vi "CMD_Drive.vi"(1 "Line":string) -> (0 "Done":bool)   [LabVIEW 2016]
uses:
  Robot Global Data.vi
  <vilib>/addons/control/pid/pid.llb/PID (DBL).vi
  <vilib>/addons/control/pid/NI_PID_pid.lvlib
  Apple Gyro/Apple Pi Gyro Library.lvlib
panel:
  in  "Subcommands":string[](array[string])=["at", "at", "for", "to", "until"]
  in  "Parameters":i32[](array[numeric])=[1, 3, 3, 3, 1]
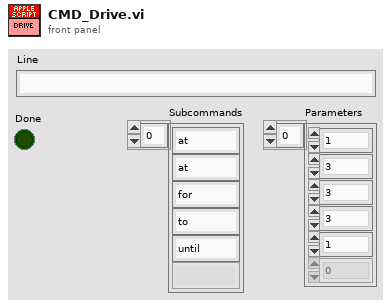
[diagram p1: front panel]
types:
  T1 = cluster{"proportional gain (Kc)":dbl, "integral time (Ti, min)":dbl, "derivative time (Td, min)":dbl}
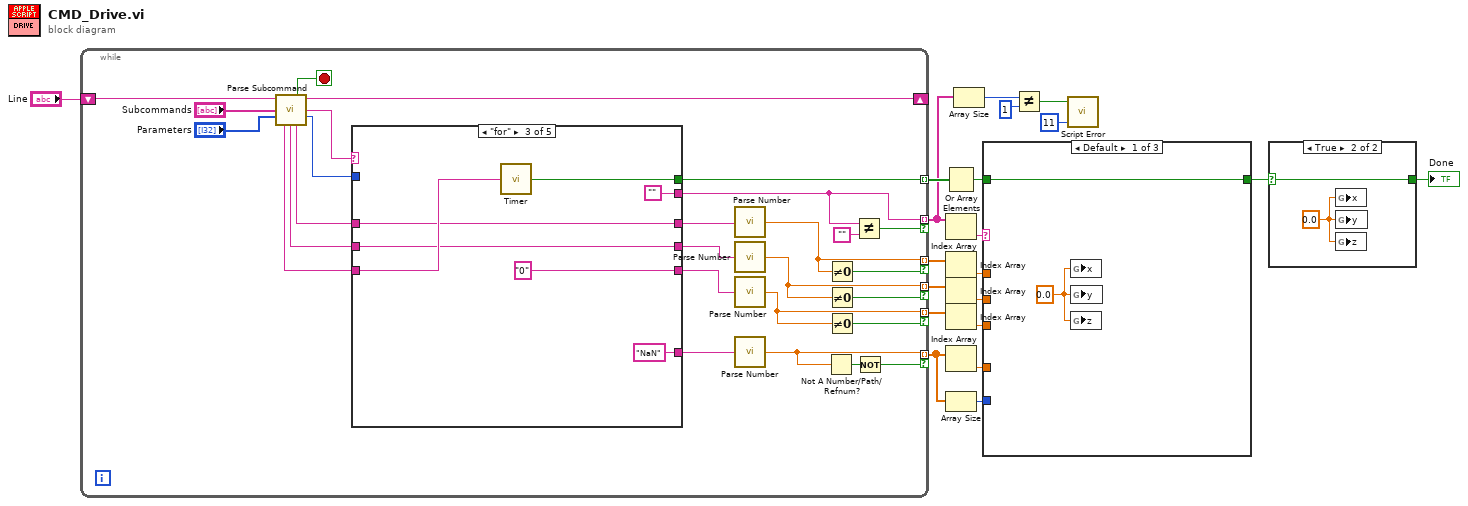
[diagram p0: block diagram]
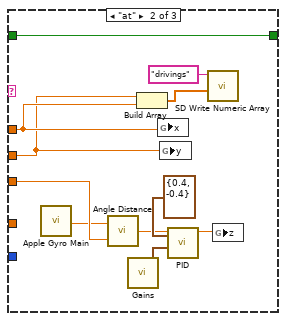
[diagram p3: hidden frame]
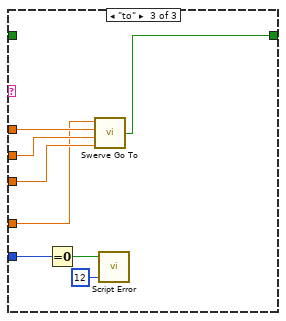
[diagram p4: hidden frame]
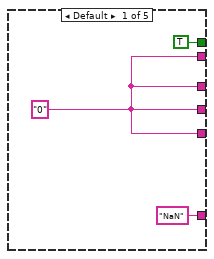
[diagram p5: hidden frame]
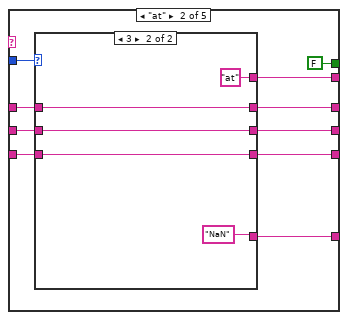
[diagram p6: hidden frame]
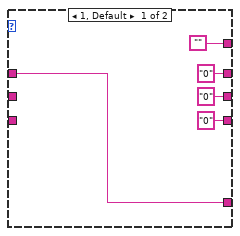
[diagram p7: hidden frame]
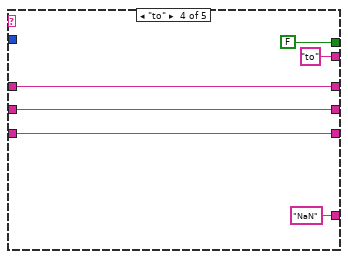
[diagram p8: hidden frame]
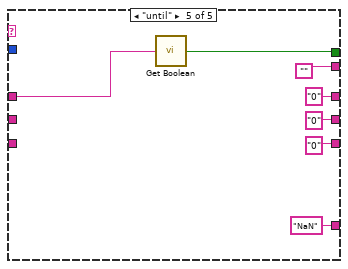
[diagram p9: hidden frame]
diagram:
  n1 = while {
    shift-right: [w44] -> _
    shift-left: "Line" -> [w47]
    tunnel: [w21] -> w5 mode=indexing
    tunnel: [w33] -> w17 mode=indexing if=w27
    tunnel: [w32] -> w15 mode=indexing if=w25
    tunnel: [w29] -> w13 mode=indexing if=w26
    tunnel: [w24] -> w3 mode=indexing if=w22
    tunnel: [w35] -> w4 mode=indexing if=w36
    stop <- w43 stop-if-true
    n2 = call "Parse Subcommand.vi"("Text In"=w47, "Subcommands"="Subcommands", "Parameters"="Parameters") -> ("Done"=w43:bool, "Text Out"=w44:string, "Subcommand"=w42:string, "# of Parameters"=w41:i32, "Parameter 3"=w39:string, "Parameter 2"=w38:string, "Parameter 1"=w40:string)  [unwired: 6 in]
    n3 = case shown="\"for\"" w42 {
      tunnel: w41 -> [_ w60 _ _ _]
      tunnel: w40 -> [_ w59 w72 w83 w85]
      tunnel: w38 -> [_ w58 w71 w82 _]
      tunnel: w39 -> [_ w57 w73 w81 _]
      tunnel: [w49 w56 w72 w83 "0" ("Parameter 1")] -> w34
      tunnel: [w49 w55 w71 w82 "0" ("Parameter 1")] -> w31
      tunnel: [w49 w54 "0" ("Parameter 3") w81 "0" ("Parameter 1")] -> w30
      tunnel: [TRUE ("Value") FALSE ("Running") w74 FALSE w84] -> w21
      tunnel: [w49 w51 "" "to" ("format string") ""] -> w35
      tunnel: ["NaN" ("Parameter 1") w53 "NaN" ("Parameter 3") "NaN" ("Parameter 3") "NaN" ("Parameter 1")] -> w28
      frame Default {
        w49 = "0" ("format string")
      }
      frame "at" {
        n4 = case shown="3" w60 {
          tunnel: w59 -> [w63 w70]
          tunnel: w58 -> [_ w69]
          tunnel: w57 -> [_ w66]
          tunnel: ["0" ("Parameter 2") w70] -> w56
          tunnel: ["0" ("Parameter 2") w69] -> w55
          tunnel: ["0" ("Parameter 3") w66] -> w54
          tunnel: [w63 "NaN" ("Parameter 3")] -> w53
          tunnel: ["" "at"] -> w51
          frame 1, Default {
          }
          frame 3 {
          }
        }
      }
      frame "for" {
        n5 = call "Timer.vi"("Seconds (string)"=w73) -> ("Done"=w74:bool)
      }
      frame "to" {
      }
      frame "until" {
        n6 = call "Get Boolean.vi"("Name"=w85) -> ("Value"=w84:bool)
      }
    }
    n7 = call "Parse Number.vi"("String"=w34) -> ("Number"=w33:dbl)
    n8 = call "Parse Number.vi"("String"=w31) -> ("Number"=w32:dbl)
    n9 = call "Parse Number.vi"("String"=w30) -> ("Number"=w29:dbl)
    n10 = call "Parse Number.vi"("String"=w28) -> ("Number"=w24:dbl)
    n11 = Not A Number/Path/Refnum?(number/path/refnum=w24) -> (NaN/Path/Refnum?=w23:bool)
    n12 = Not Equal To 0?(x=w33) -> (x != 0?=w27:bool)
    n13 = Not Equal To 0?(x=w32) -> (x != 0?=w25:bool)
    n14 = Not Equal To 0?(x=w29) -> (x != 0?=w26:bool)
    n15 = Not Equal?(x=w35, y="") -> (x != y?=w36:bool)
    n16 = Not(x=w23) -> (.not. x?=w22:bool)
  }
  n17 = Or Array Elements(Boolean array=w5) -> (logical OR=w1:bool)
  n18 = Index Array(array=w4) -> (element=w10:string)  [unwired: 1 in]
  n19 = Index Array(array=w17) -> (element=w16:dbl)  [unwired: 1 in]
  n20 = Index Array(array=w15) -> (element=w14:dbl)  [unwired: 1 in]
  n21 = Index Array(array=w13) -> (element=w12:dbl)  [unwired: 1 in]
  n22 = Index Array(array=w3) -> (element=w11:dbl)  [unwired: 1 in]
  n23 = Array Size(array=w3) -> (size(s)=w2:i32)
  n24 = Array Size(array=w4) -> (size(s)=w8:i32)
  n25 = case shown="Default" w10 {
    tunnel: w16 -> [_ w95 w111]
    tunnel: w1 -> [w92 w103 _]
    tunnel: [w92 w103 w104] -> w18
    tunnel: w14 -> [_ w94 w110]
    tunnel: w12 -> [_ w98 w109]
    tunnel: w11 -> [_ _ w108]
    tunnel: w2 -> [_ _ w106]
    frame Default {
      w91 = 0.0 ("X")
      n26 = global write "Robot Global Data.vi" "x"(w91) -> ()
      n27 = global write "Robot Global Data.vi" "y"(w91) -> ()
      n28 = global write "Robot Global Data.vi" "z"(w91) -> ()
    }
    frame "at" {
      n29 = call "Apple Gyro Main.vi"() -> ("Gyro Yaw Out"=w97:dbl)  [unwired: 4 in]
      n30 = call "Angle Distance.vi"("target angle"=w98, "current angle"=w97) -> ("distance"=w99:dbl)
      n31 = call "Gains.vi"() -> ("Rot"=w96:T1)  [unwired: 10 in, 1 out]
      n32 = Build Array(w94, w95) -> (w100:dbl[])
      n33 = global write "Robot Global Data.vi" "x"(w95) -> ()
      n34 = global write "Robot Global Data.vi" "y"(w94) -> ()
      n35 = call-poly <vilib>:"PID.vi"("output range"=cluster{"output high":dbl, "output low":dbl} {"output high"=0.4, "output low"=-0.4}, "PID gains"=w96, "setpoint"=w99) -> ("output"=w93:dbl)  [unwired: 7 in, 1 out]
      n36 = call <vilib>:"SD Write Numeric Array.vi"("Numeric Array"=w100, "Name"="drivings") -> ()  [unwired: 8 in, 2 out]
      n37 = global write "Robot Global Data.vi" "z"(w93) -> ()
    }
    frame "to" {
      n38 = Equal To 0?(x=w106) -> (x = 0?=w105:bool)
      n39 = call "Swerve Go To.vi"("Max Speed"=w108, "Target X"=w111, "Target Y"=w110, "Target Angle"=w109) -> ("Done"=w104:bool)  [unwired: 3 in]
      n40 = call "Script Error.vi"("Error?"=w105, "Error Code"=12) -> ()  [unwired: 3 in, 1 out]
    }
  }
  n41 = Not Equal?(x=w8, y=1) -> (x != y?=w6:bool)
  n42 = call "Script Error.vi"("Error?"=w6, "Error Code"=11) -> ()  [unwired: 3 in, 1 out]
  n43 = case shown="True" w18 {
    selector: w18 -> [w112 w114]
    tunnel: [w112 w114] -> w19
    frame False {
    }
    frame True {
      w113 = 0.0 ("X")
      n44 = global write "Robot Global Data.vi" "x"(w113) -> ()
      n45 = global write "Robot Global Data.vi" "y"(w113) -> ()
      n46 = global write "Robot Global Data.vi" "z"(w113) -> ()
    }
  }
  "Done" <- w19
